vi "Make_data_file.vi"(1 "File Name":string) -> (0 "File Refnum":refnum<file>)   [LabVIEW 2016]
panel:
  in  "Error In":errorcluster
  out "Error Out":errorcluster
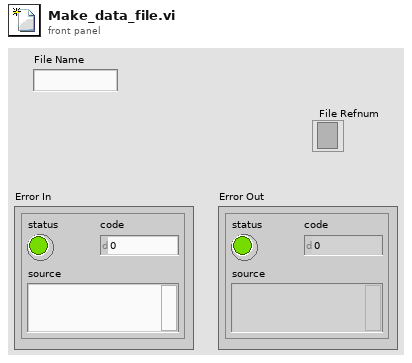
[diagram p1: front panel]
types:
  T1 = enum16{"open", "replace", "create", "open or create", "replace or create", "replace or create with confirmation"}
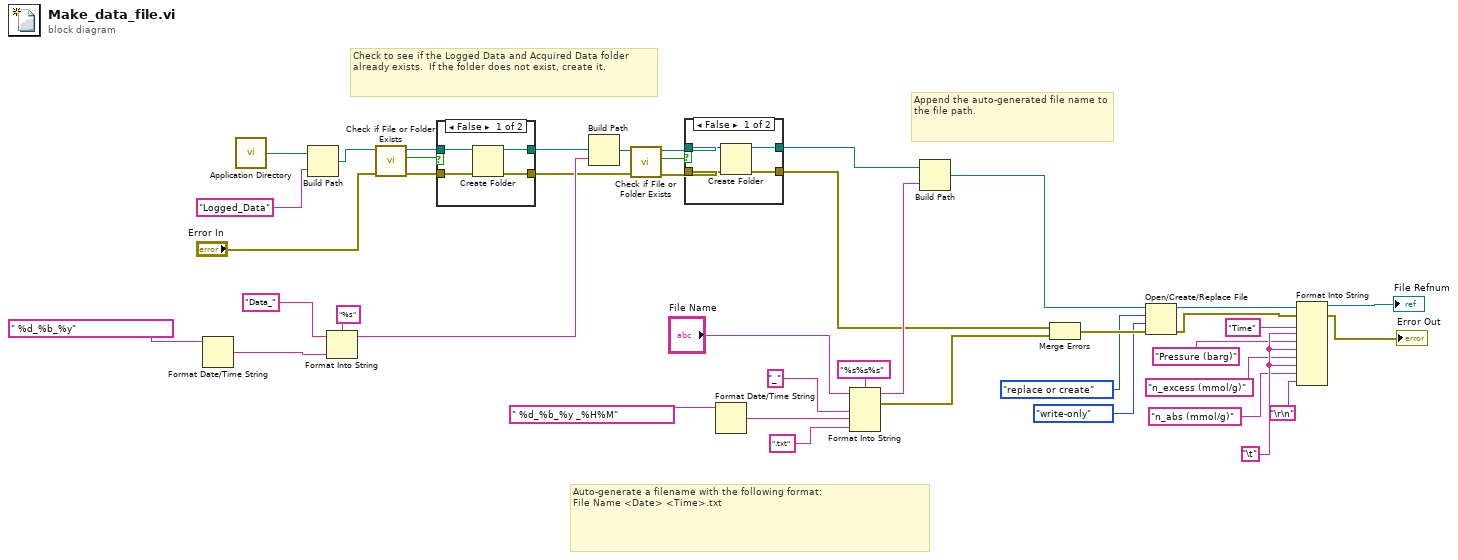
[diagram p0: block diagram]
diagram:
  w9 = "\t"
  # "Append the auto-generated file name to the file path."
  # "Check to see if the Logged Data and Acquired Data folder already exists.  If the folder does not exist, create it."
  # "Auto-generate a filename with the following format:\nFile Name <Date> <Time>.txt"
  n1 = Format Date/Time String(time format string (%c)=" %d_%b_%y") -> (date/time string=w24:string)  [unwired: 2 in]
  n2 = call <vilib>:"Application Directory.vi"() -> ("Application Directory"=w32:path)
  n3 = Build Path(base path=w32, name or relative path="Logged_Data" ("prompt (Create Folder)")) -> (appended path=w36:path)
  n4 = Format Into String(format string="%s", initial string="Data_" ("string"), w24) -> (resulting string=w22:string)  [unwired: 1 in, 1 out]
  n5 = call <vilib>:"Check if File or Folder Exists.vi"("error in (no error)"="Error In", "path"=w36) -> ("error out"=w35:errorcluster, "file or folder exists?"=w33:bool, "dup path"=w34:path)  [unwired: 7 in]
  n6 = case shown="False" w33 {
    tunnel: [w46 w48] -> w27
    tunnel: [w45 w47] -> w21
    tunnel: w35 -> [w44 w47]
    tunnel: w34 -> [w43 w48]
    frame False {
      n7 = Create Folder(path (use dialog)=w43, error in=w44) -> (created path=w46:path, error out=w45:errorcluster)  [unwired: 1 in, 1 out]
    }
    frame True {
    }
  }
  n8 = Build Path(base path=w27, name or relative path=w22) -> (appended path=w20:path)
  n9 = call <vilib>:"Check if File or Folder Exists.vi"("error in (no error)"=w21, "path"=w20) -> ("error out"=w17:errorcluster, "file or folder exists?"=w18:bool, "dup path"=w19:path)  [unwired: 7 in]
  n10 = case shown="False" w18 {
    tunnel: [w52 w54] -> w16
    tunnel: [w51 w53] -> w15
    tunnel: w17 -> [w50 w53]
    tunnel: w19 -> [w49 w54]
    frame False {
      n11 = Create Folder(path (use dialog)=w49, error in=w50) -> (created path=w52:path, error out=w51:errorcluster)  [unwired: 1 in, 1 out]
    }
    frame True {
    }
  }
  n12 = Format Date/Time String(time format string (%c)=" %d_%b_%y _%H%M") -> (date/time string=w13:string)  [unwired: 2 in]
  n13 = Format Into String(format string="%s%s%s", initial string="File Name", "_" ("input 1"), w13, ".txt" ("string")) -> (resulting string=w28:string, error out=w29:errorcluster)  [unwired: 1 in]
  n14 = Build Path(base path=w16, name or relative path=w28) -> (appended path=w42:path)
  n15 = Merge Errors(w15, w29) -> (w41:errorcluster)
  n16 = Open/Create/Replace File(file path (use dialog)=w42, error in=w41, operation (0:open)=T1."replace or create", access (0:read/write)=enum16{"read/write", "read-only", "write-only"}."write-only") -> (refnum out=w10:refnum<file>, error out=w2:errorcluster)  [unwired: 2 in, 1 out]
  n17 = Format Into String(initial string=w10, error in=w2, "Time", w9, "Pressure (barg)", w9, "n_excess (mmol/g)", w9, "n_abs (mmol/g)" ("input 7"), "\r\n") -> (resulting string=→"File Refnum":refnum<file>, error out=→"Error Out":errorcluster)  [unwired: 1 in]
